vi "Evaluate Boolean Shared Variable.vi"(6 "error in (no error)":errorcluster, 7 "Access":T1=enum."Read", 8 "Read Values":dbl[](array[numeric]), 9 "Boolean Array Index":i32[](array[numeric]), 10 "Boolean Array":refnum<k21>[](array[refnum]), 11 "Write Values in":dbl[](array[numeric])) -> (0 "error out":errorcluster, 3 "Write Values out":dbl[](array[numeric]))   [LabVIEW 2012, in "Shared Variable Custom Device.lvlib"]
uses:
  Shared Variable Custom Device.lvlib
  Shared Variable/Shared Variable Access.ctl
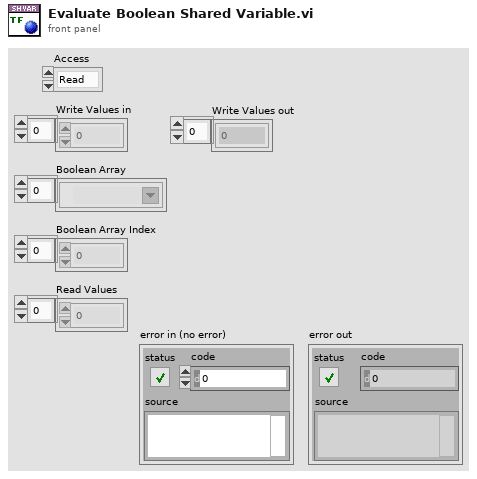
[diagram p1: front panel]
types:
  T1 = typedef "Shared Variable Custom Device.lvlib/Shared Variable Access.ctl" = enum16{"Write", "Read"}
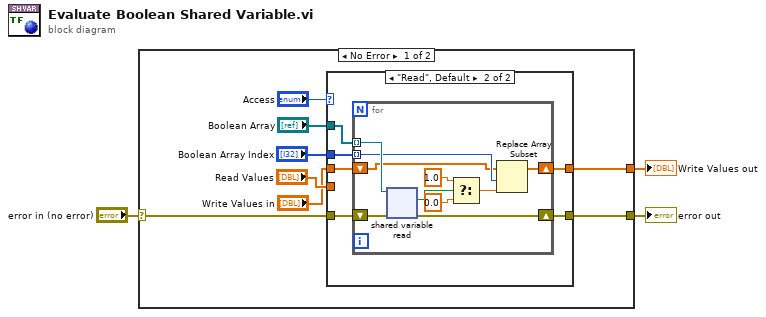
[diagram p0: block diagram]
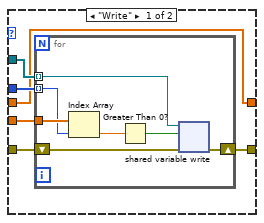
[diagram p2: hidden frame]
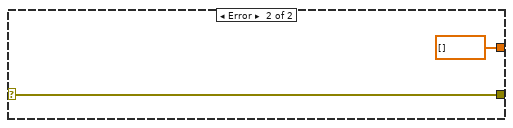
[diagram p3: hidden frame]
diagram:
  n1 = case shown="No Error" "error in (no error)" {
    selector: "error in (no error)" -> [w5 w42]
    tunnel: [w6 dbl[] [] ("Write Values in")] -> w3
    tunnel: [w4 w42] -> w1
    frame No Error {
      n2 = case shown="\"Read\", Default" "Access" {
        tunnel: "Read Values" -> [w17 _]
        tunnel: "Boolean Array Index" -> [w16 w30]
        tunnel: "Boolean Array" -> [w15 w29]
        tunnel: "Write Values in" -> [w14 w28]
        tunnel: [w14 w27] -> w6
        tunnel: w5 -> [w13 w26]
        tunnel: [w12 w25] -> w4
        frame "Write" {
          n3 = for {
            tunnel: w15 -> [w24] mode=indexing
            tunnel: w17 -> [w23]
            tunnel: w16 -> [w22] mode=indexing
            shift-right: [w18] -> w12
            shift-left: w13 -> [w19]
            n4 = Index Array(array=w23, index=w22) -> (element=w21:dbl)
            n5 = Greater Than 0?(x=w21) -> (x > 0?=w20:bool)
            n6 = shared-variable-write(w24, w19, w20) -> (w18:errorcluster)  [unwired: 1 out]
          }
        }
        frame "Read", Default {
          n7 = for {
            tunnel: w29 -> [w40] mode=indexing
            shift-right: [w37] -> w27
            shift-left: w28 -> [w38]
            tunnel: w30 -> [w39] mode=indexing
            shift-right: [w31] -> w25
            shift-left: w26 -> [w32]
            n8 = shared-variable-read(w40, w32) -> (w31:errorcluster, w36:bool)  [unwired: 2 out]
            n9 = Select(t=1.0, s=w36, f=0.0) -> (s? t:f=w33:dbl)
            n10 = Replace Array Subset(array=w38, new element=w33, index=w39) -> (w37:dbl[])
          }
        }
      }
    }
    frame Error {
    }
  }
  "Write Values out" <- w3
  "error out" <- w1
